vi "Actor Core.vi"(8 "error in":errorcluster, 11 "Digital Reader in":refnum<class "Digital Reader.lvclass">) -> (0 "error out":errorcluster, 3 "Actor out":refnum<class "Actor.lvclass">)   [LabVIEW 2024, in "DAQmx Actor.lvlib" / "Digital Reader.lvclass"]
doc: "<p>(<strong>Filename</strong>: <span class=\"dnl\">Actor Framework.lvlib:Actor.lvclass:Actor Core.vi</span>)</p>\n<p>Receives messages to the actor, reacts to them, and initiates any error handling that may shut the actor down.</p>\n<p>Descendant classes may override this VI to append parallel tasks for the actor to complete while it handles messages. Overrides use the <a href=\"nihelplauncher://docs/csh?context=lvcore_glang_udclass\">Call Parent Class Method</a> node.</p>"
uses:
  Digital Reader.lvclass
  C:/Users/ottoa/OneDrive/Desktop/working copies/DAQmxActor/src/DAQmx Actor/DAQmx Actor/DAQmx Actor.lvclass
  C:/Program Files (x86)/National Instruments/LabVIEW 2024/vi.lib/ActorFramework/Actor/Actor.lvclass
  <vilib>/ActorFramework/Actor/Actor.lvclass
  <vilib>/ActorFramework/Actor/Actor.lvclass/Actor.ctl
  Digital Reader.lvclass/Digital Reader.ctl
  DAQmx Actor Interface/DAQmx Actor Interface Messages/Digital Input Data Msg/Digital Input Data Msg.lvclass/Digital Input Data Msg.ctl
  <vilib>/ActorFramework/Message Enqueuer/Message Enqueuer.lvclass/Message Enqueuer.ctl
  <vilib>/DAQmx/read.llb/DAQmx Read (Digital 1D Bool NChan 1Samp 1Line).vi
  <vilib>/ActorFramework/Message Enqueuer/Enqueue.vi
  DAQmx Actor Interface/DAQmx Actor Interface Messages/Digital Input Data Msg/Digital Input Data Msg.lvclass
  C:/Program Files (x86)/National Instruments/LabVIEW 2024/vi.lib/ActorFramework/Message/Message.lvclass
  <vilib>/DAQmx/miscellaneous.llb/DAQmx Fill In Error Info.vi
  <vilib>/ActorFramework/Message Priority Queue/Priority Enqueue.vi
  DAQmx Actor/DAQmx Actor.lvclass
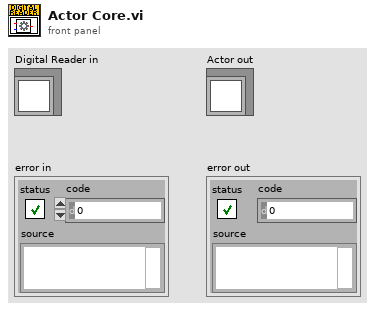
[diagram p1: front panel]
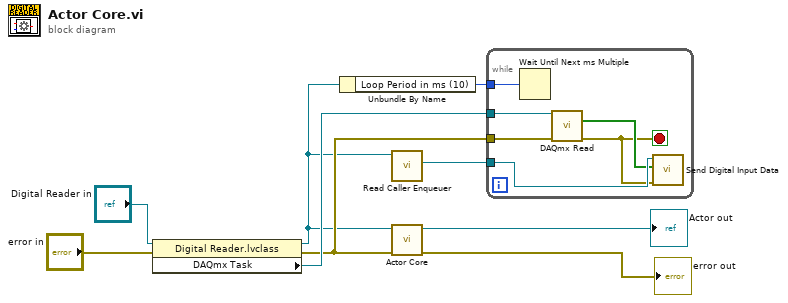
[diagram p0: block diagram]
diagram:
  n1 = property class="Digital Reader.lvclass"(reference="Digital Reader in", error in="error in") -> (reference out=w2:refnum<class "Digital Reader.lvclass">, error out=w3:errorcluster, "DAQmx Task"=w6:refnum<k21>)
  n2 = Unbundle By Name(w2) -> ("Loop Period in ms (10)"=w5:u32)
  n3 = call <vilib>:"Read Caller Enqueuer.vi"("Actor"=w2) -> ("Caller Enqueuer"=w1:refnum<class "Message Enqueuer.lvclass">)  [unwired: 10 in]
  n4 = call-parent "Actor Core.vi"("error in"=w3, "Actor in"=w2) -> ("error out"=→"error out":errorcluster, "Actor out"=→"Actor out":refnum<class "Actor.lvclass">)  [unwired: 8 in]
  n5 = while {
    tunnel: w6 -> [w15]
    tunnel: w5 -> [w14]
    tunnel: w3 -> [w13]
    tunnel: w1 -> [w12]
    stop <- w10 stop-if-true
    n6 = Wait Until Next ms Multiple(millisecond multiple=w14) -> ()  [unwired: 1 out]
    n7 = call-poly <vilib>:"DAQmx Read.vi"("task/channels in"=w15, "error in"=w13) -> ("data"=w11:bool[], "error out"=w10:errorcluster)  [unwired: 11 in, 1 out]
    n8 = call "Send Digital Input Data.vi"("error in (no error)"=w10, "Digital Data"=w11, "Message Enqueuer"=w12) -> ()  [unwired: 7 in, 2 out]
  }
